vi "BiasSpectroscopySetTimeConstant.vi"(2 "Set Time Constant":T1(ring)=enum."10 ms", 3 "Application ref in":refnum<vi>) -> (1 "Application ref out":refnum<vi>)   [LabVIEW 2021]
uses:
  <userlib>/Nanonis Prog Interface V5/Nanonis Prog Interface.lvlib
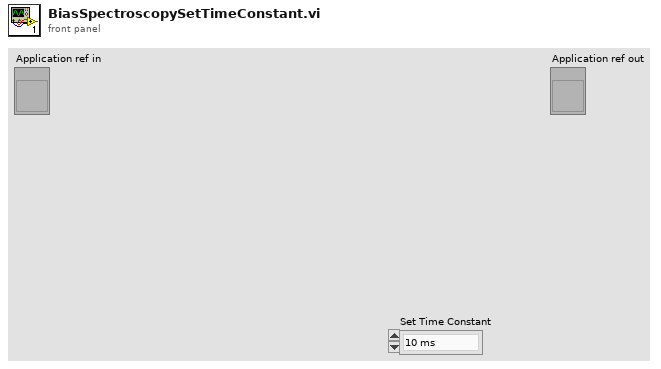
[diagram p1: front panel]
types:
  T1 = enum16{"10 us", "30 us", "100 us", "300 us", "1 ms", "3 ms", "10 ms", "30 ms", "100 ms", "300 ms", "1 s", "3 s", "10 s", "30 s", "100 s", "300 s", "1 ks", "3 ks", "10 ks", "30 ks"}
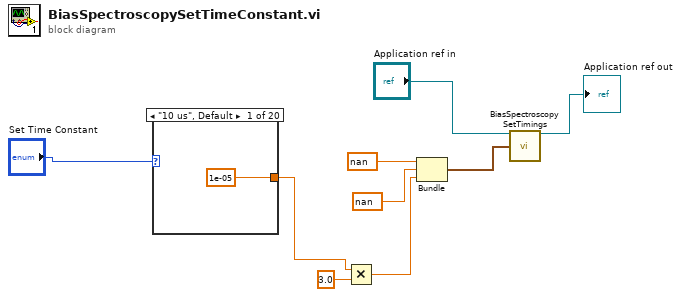
[diagram p0: block diagram]
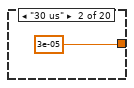
[diagram p2: hidden frame]
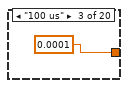
[diagram p3: hidden frame]
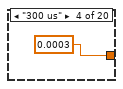
[diagram p4: hidden frame]
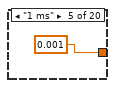
[diagram p5: hidden frame]
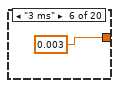
[diagram p6: hidden frame]
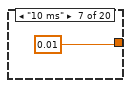
[diagram p7: hidden frame]
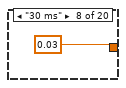
[diagram p8: hidden frame]
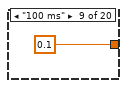
[diagram p9: hidden frame]
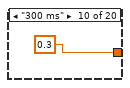
[diagram p10: hidden frame]
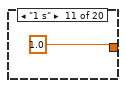
[diagram p11: hidden frame]
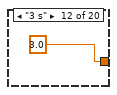
[diagram p12: hidden frame]
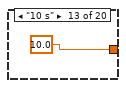
[diagram p13: hidden frame]
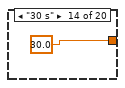
[diagram p14: hidden frame]
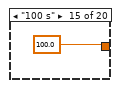
[diagram p15: hidden frame]
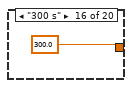
[diagram p16: hidden frame]
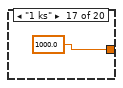
[diagram p17: hidden frame]
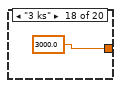
[diagram p18: hidden frame]
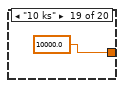
[diagram p19: hidden frame]
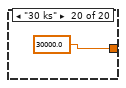
[diagram p20: hidden frame]
diagram:
  n1 = case shown="\"10 us\", Default" "Set Time Constant" {
    tunnel: [1e-05 3e-05 0.0001 0.0003 0.001 0.003 0.01 0.03 0.1 0.3 1.0 3.0 10.0 30.0 100.0 300.0 1000.0 3000.0 10000.0 30000.0] -> w6
    frame "10 us", Default {
    }
    frame "30 us" {
    }
    frame "100 us" {
    }
    frame "300 us" {
    }
    frame "1 ms" {
    }
    frame "3 ms" {
    }
    frame "10 ms" {
    }
    frame "30 ms" {
    }
    frame "100 ms" {
    }
    frame "300 ms" {
    }
    frame "1 s" {
    }
    frame "3 s" {
    }
    frame "10 s" {
    }
    frame "30 s" {
    }
    frame "100 s" {
    }
    frame "300 s" {
    }
    frame "1 ks" {
    }
    frame "3 ks" {
    }
    frame "10 ks" {
    }
    frame "30 ks" {
    }
  }
  n2 = Multiply(x=w6, y=3.0) -> (x*y=w5:dbl)
  n3 = Bundle(nan, nan, w5) -> (w1:cluster{dbl, dbl, dbl})  [unwired: 1 in]
  n4 = call <userlib>:"BiasSpectroscopy SetTimings.vi"("Application ref in"="Application ref in", "Sweep Timing (NaN)"=w1) -> ("Application ref out"=→"Application ref out":refnum<vi>)  [unwired: 12 in, 1 out]
